vi "Serialize an Object with Type Information (Inline).vi"() -> ()   [LabVIEW 2017]
doc: "Demonstrates the JSONtext Object Serializer by serializing a LabVIEW Object to JSON with inline type information."
uses:
  Generic Object Serializer/Generic Object Serializer.lvclass
  C:/Program Files (x86)/National Instruments/LabVIEW 2017/vi.lib/JDP Science/JSONtext/LVClass Serializer/JSONtext LVClass Serializer.lvclass
  Generic Object Serializer/Type Name Handling.ctl
  Generic Object Serializer/Generic Object Serializer.lvclass/Generic Object Serializer.ctl
  585c77a6-94ca-412b-a7e9-3a1ed3474501.vi
  Generic Object Serializer/Write Type Name Handling.vi
  <vilib>/JDP Science/JSONtext/Variant to JSON Text.vi
  Account/Account.lvclass
panel:
  in  "CreatedDate":timestamp=timestamp(3700276200 s since 1904-01-01)
  in  "Active":bool=TRUE
  in  "Email":string="john.doe@example.com"
  in  "Roles":string[](array[string])=["User", "Admin"]
  out "error out":errorcluster
  out "<JSON>":string
  # "Overview\nDemonstrates the JSONtext Object Serializer by serializing a LabVIEW Object to JSON with inline type information.\n\nInstructions\nRun the VI"
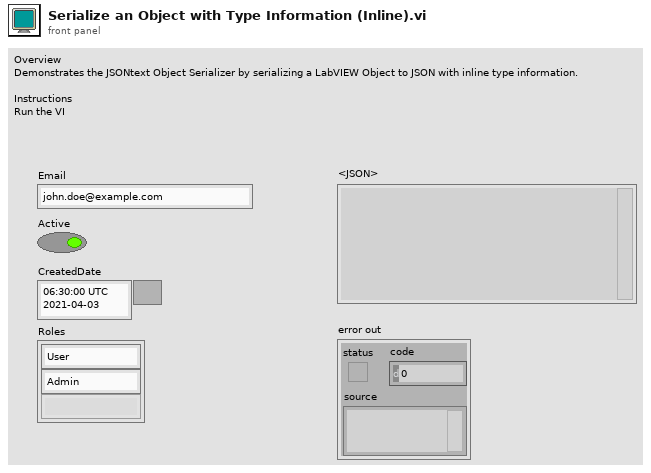
[diagram p1: front panel]
types:
  T1 = typedef "Generic Object Serializer.lvclass/Type Name Handling.ctl" = enum16{"None", "Inline"}
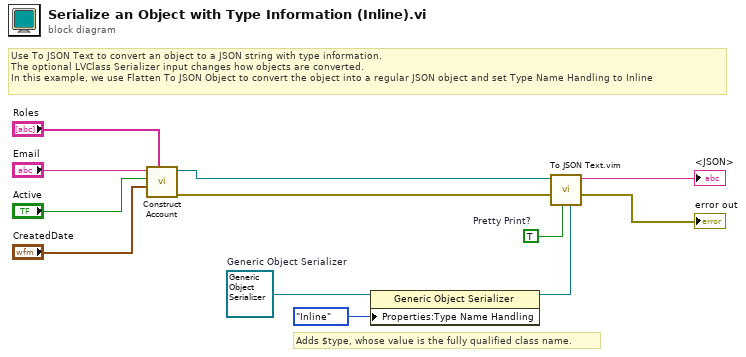
[diagram p0: block diagram]
diagram:
  w5 = refnum<class "Generic Object Serializer.lvclass"> refnum  # Generic Object Serializer
  w6 = TRUE  # Pretty Print?
  # "Adds $type, whose value is the fully qualified class name."
  # "Use To JSON Text to convert an object to a JSON string with type information.\nThe optional LVClass Serializer input changes how objects are converted.\nIn this example, we use Flatten To JSON Object to convert the object into a regular JSON object and set Type Name Handling to Inline"
  n1 = call "Construct Account.vi"("Roles"="Roles", "CreatedDate"="CreatedDate", "Active"="Active", "Email"="Email") -> ("error out"=w8:errorcluster, "Account"=w7:refnum<class "Account.lvclass">)  [unwired: 6 in]
  n2 = property class="Generic Object Serializer"(reference=w5, "Properties:Type Name Handling"=Type_Name_Handling."Inline" ("Type Name Handling")) -> (reference out=w2:refnum<class "Generic Object Serializer.lvclass">)  [unwired: 1 in, 1 out]
  n3 = call "To JSON Text.vim"("LVClass Serializer"=w2, "Pretty Print?"=w6, "error in (no error)"=w8, "Anything"=w7) -> ("error out"=→"error out":errorcluster, "<JSON>"=→"<JSON>":string)  [unwired: 6 in]
